vi "Configure Trace (Power Meter).vi"(6 "Y Scale Value (2E-8 seconds)":dbl=2e-08, 7 "Y Max Value (0 dBm)":dbl, 8 "error in (no error)":errorcluster, 9 "X Scale Time (2E-8 seconds)":dbl=2e-08, 10 "X Start Time (0 seconds)":dbl, 11 "VISA resource name":refnum<visa-resource-name>) -> (0 "error out":errorcluster, 3 "VISA resource name out":refnum<visa-resource-name>)   [LabVIEW 2022 SP3, in "Agilent N934X Series.lvlib"]
doc: "Configures the trace setting of Power Meter Measurement Type.\n\nNote:\nThis VI is only applicable for N9321C, N9322C, N9323C, N9324C models."
uses:
  <instrlib>/Agilent N934X Series/Agilent N934X Series.lvlib
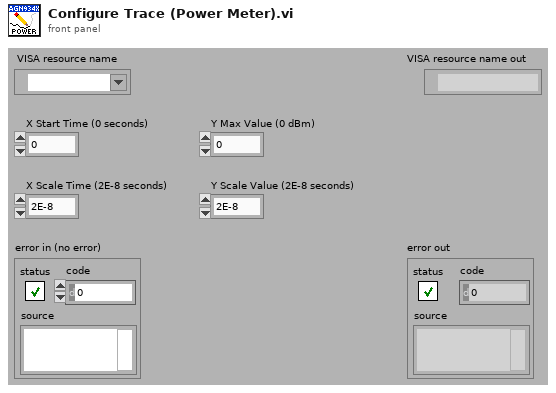
[diagram p1: front panel]
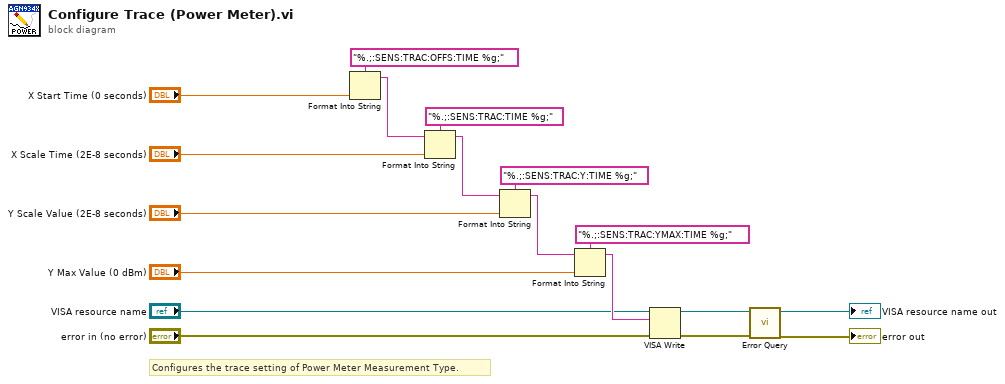
[diagram p0: block diagram]
diagram:
  # "Configures the trace setting of Power Meter Measurement Type."
  n1 = Format Into String(format string="%.;:SENS:TRAC:OFFS:TIME %g;", "X Start Time (0 seconds)") -> (resulting string=w16:string)  [unwired: 2 in, 1 out]
  n2 = Format Into String(format string="%.;:SENS:TRAC:TIME %g;", initial string=w16, "X Scale Time (2E-8 seconds)") -> (resulting string=w13:string)  [unwired: 1 in, 1 out]
  n3 = Format Into String(format string="%.;:SENS:TRAC:Y:TIME %g;", initial string=w13, "Y Scale Value (2E-8 seconds)") -> (resulting string=w10:string)  [unwired: 1 in, 1 out]
  n4 = Format Into String(format string="%.;:SENS:TRAC:YMAX:TIME %g;", initial string=w10, "Y Max Value (0 dBm)") -> (resulting string=w7:string)  [unwired: 1 in, 1 out]
  n5 = VISA Write(VISA resource name="VISA resource name", write buffer=w7, error in (no error)="error in (no error)") -> (VISA resource name out=w4:refnum<visa-resource-name>, error out=w3:errorcluster)  [unwired: 1 out]
  n6 = call <instrlib>:"Error Query.vi"("error in (no error)"=w3, "VISA resource name"=w4) -> ("error out"=→"error out":errorcluster, "VISA resource name out"=→"VISA resource name out":refnum<visa-resource-name>)  [unwired: 6 in, 2 out]
